vi "Write Verification Depth.vi"(8 "error in (no error)":errorcluster, 10 "Verification Depth":i32=4, 11 "SSL Client Context in":refnum<class "SSL Client Context.lvclass">) -> (0 "error out":errorcluster, 3 "SSL Client Context out":refnum<class "SSL Client Context.lvclass">)   [LabVIEW 2013, in "OpenSSL Socket.lvlib" / "SSL Client Context.lvclass"]
uses:
  SSL Client Context.lvclass
  SSL Client Context.lvclass/SSL Client Context.ctl
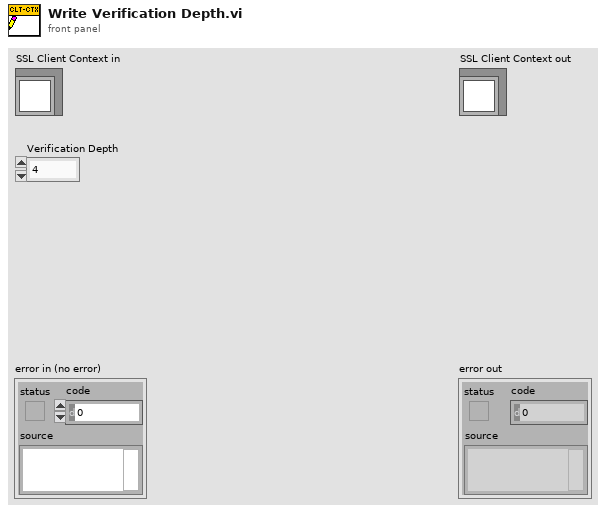
[diagram p1: front panel]
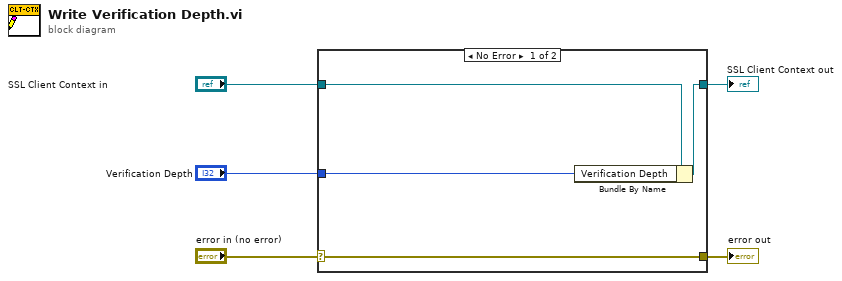
[diagram p0: block diagram]
diagram:
  n1 = case shown="No Error" "error in (no error)" {
    selector: "error in (no error)" -> [w9 w10]
    tunnel: [w9 w10] -> w4
    tunnel: [w7 w11] -> w2
    tunnel: "SSL Client Context in" -> [w8 w11]
    tunnel: "Verification Depth" -> [w6 _]
    frame No Error {
      n2 = Bundle By Name(cluster=w8, "Verification Depth"=w6) -> (w7:refnum<class "SSL Client Context.lvclass">)
    }
    frame Error {
    }
  }
  "error out" <- w4
  "SSL Client Context out" <- w2
